vi "Operator.vi"(8 "error in (no error)":errorcluster, 11 "Binary Operator in":refnum<class "Binary Operator.lvclass">) -> (0 "error out":errorcluster, 2 "Operator":string, 3 "Binary Operator out":refnum<class "Binary Operator.lvclass">)   [LabVIEW 2017, in "Transparent Assertions.lvlib" / "Constraints.lvlib" / "Binary Operator.lvclass"]
uses:
  Binary Operator.lvclass
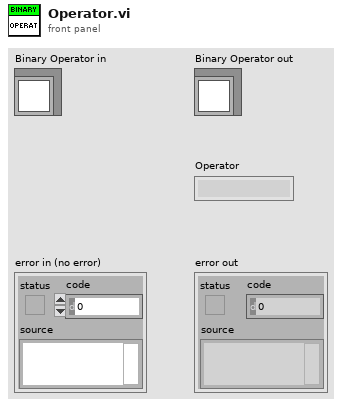
[diagram p1: front panel]
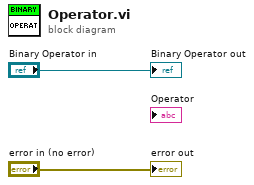
[diagram p0: block diagram]
diagram:
  "error out" <- "error in (no error)"
  "Binary Operator out" <- "Binary Operator in"
